vi "Analyze Fell Rocks.vi"(0 "Rock Position in Chamber in":i32=3, 1 "Push List":cluster{u8, i32}[](array[cluster]), 2 "Chamber":u32[][](array[colorbox]), 3 "Rock Settled ?":bool, 4 "Initialize ? (F)":bool) -> (5 "#Rocks Settled":i32, 6 "Tower Height":u64, 7 "Sequence Analysis":T1, 9 "Tower Heights":map{i32, u64}(c390))   [LabVIEW 2020, in "AoC 2022.lvlib"]
uses:
  AoC 2022.lvlib
  Sequence Analysis.ctl
  <vilib>/Utility/miscctls.llb/LVMapReplaceAction.ctl
panel:
  out "Sequence Found ? out":bool
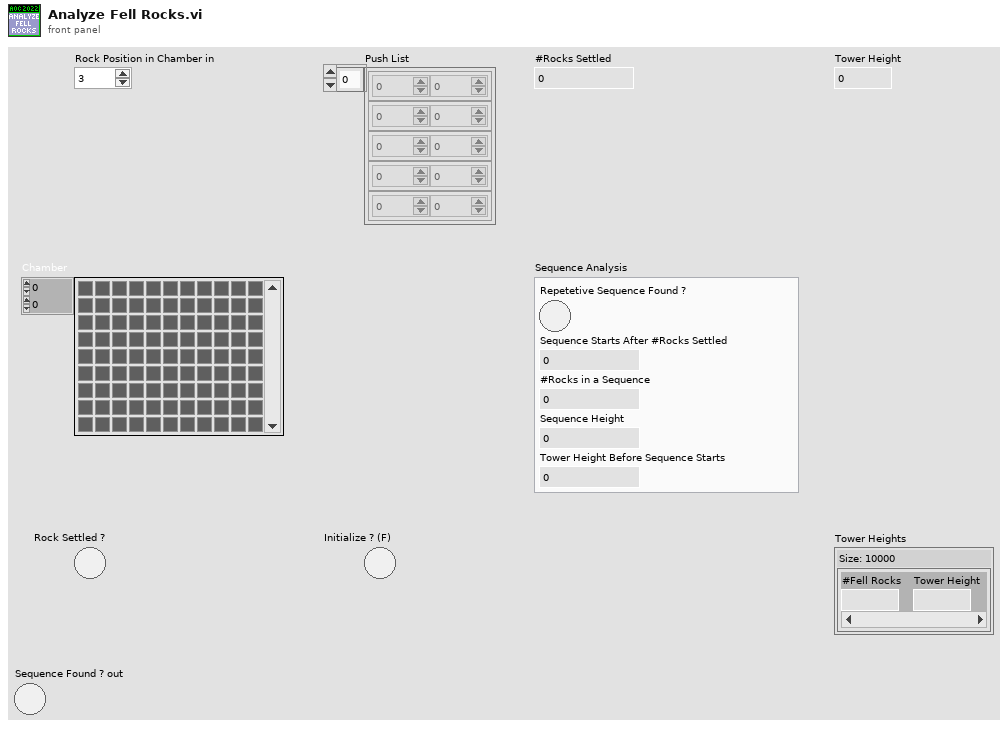
[diagram p1: front panel]
types:
  T1 = typedef "AoC 2022.lvlib/Sequence Analysis.ctl" = cluster{"Repetetive Sequence Found ?":bool, "Sequence Starts After #Rocks Settled":i32, "#Rocks in a Sequence":i32, "Sequence Height":u64, "Tower Height Before Sequence Starts":u64}
  T2 = map{cluster{"Chamber":u32[][], "Push Action":string}, i32[]}
  T3 = typedef "LVMapReplaceAction.ctl" = enum32{"Modify Entry only if found", "Add or Modify Entry", "Delete Entry"}
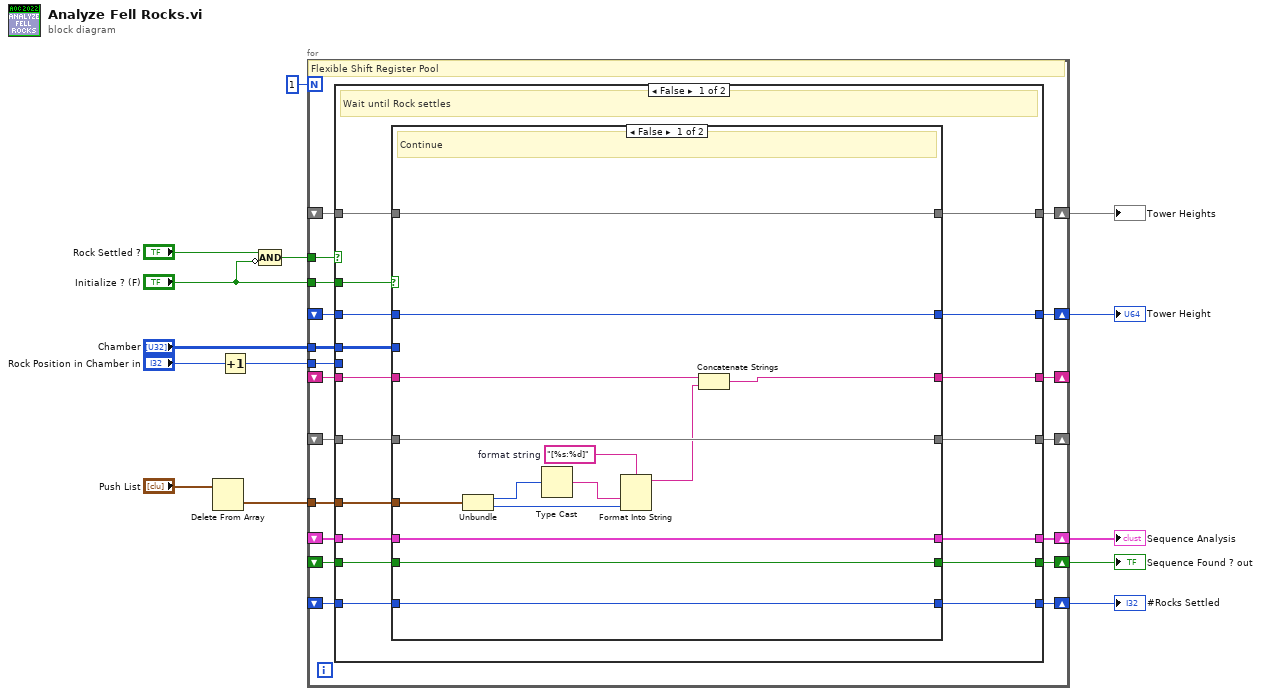
[diagram p0: block diagram]
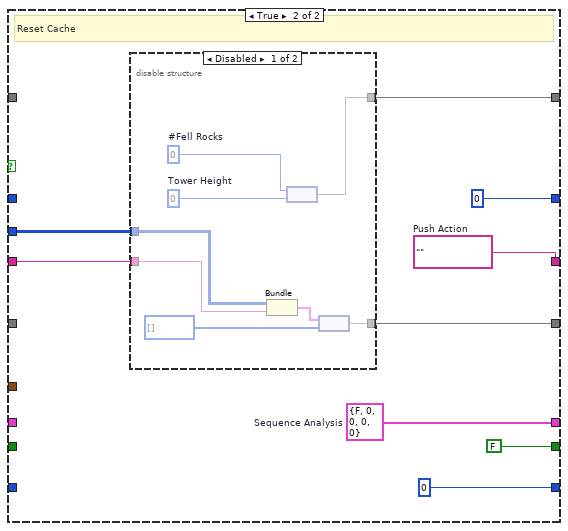
[diagram p2: hidden frame]
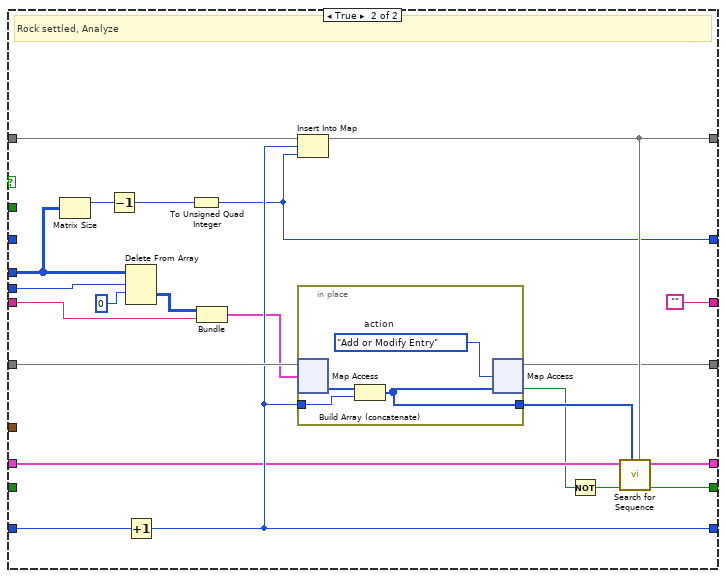
[diagram p4: hidden frame]
diagram:
  n1 = Delete From Array(array="Push List") -> (deleted portion=w6:cluster{u8, i32})  [unwired: 2 in, 1 out]
  n2 = Increment(x="Rock Position in Chamber in") -> (x+1=w4:i32)
  n3 = Compound Arithmetic op=AND("Rock Settled ?", invert "Initialize ? (F)") -> (w10:bool)
  n4 = for {
    N: 1 -> [_]
    tunnel: "Chamber" -> [w28]
    shift-right: [w29] -> _
    shift-left: _ -> [w33]
    tunnel: w10 -> [w32]
    shift-right: [w30] -> w11
    shift-left: _ -> [w31]
    tunnel: "Initialize ? (F)" -> [w27]
    shift-right: [w26] -> w3
    shift-left: _ -> [w25]
    shift-right: [w24] -> w2
    shift-left: _ -> [w23]
    shift-right: [w22] -> w9
    shift-left: _ -> [w21]
    tunnel: w6 -> [w20]
    shift-right: [w19] -> _
    shift-left: _ -> [w18]
    tunnel: w4 -> [w17]
    shift-right: [w16] -> w1
    shift-left: _ -> [w15]
    # "Flexible Shift Register Pool"
    n5 = case shown="False" w32 {
      tunnel: w33 -> [w46 w99]
      tunnel: w31 -> [w48 _]
      tunnel: [w49 w83] -> w30
      tunnel: [w47 w82] -> w29
      tunnel: w28 -> [w36 w98]
      tunnel: w27 -> [w50 _]
      tunnel: [w44 w103] -> w26
      tunnel: w25 -> [w45 w89]
      tunnel: [w42 w91] -> w24
      tunnel: w23 -> [w43 _]
      tunnel: [w41 w93] -> w22
      tunnel: w21 -> [w40 w100]
      tunnel: w20 -> [w39 _]
      tunnel: [w38 ""] -> w19
      tunnel: w18 -> [w37 w101]
      tunnel: w17 -> [_ w95]
      tunnel: [w35 w88] -> w16
      tunnel: w15 -> [w34 w94]
      frame False {
        # "Wait until Rock settles"
        n6 = case shown="False" w50 {
          tunnel: [w64 u64 0] -> w49
          tunnel: w48 -> [w64 _]
          tunnel: [w63 w65] -> w47
          tunnel: w46 -> [w63 _]
          tunnel: w45 -> [w62 _]
          tunnel: [w62 w66] -> w44
          tunnel: w43 -> [w61 _]
          tunnel: [w61 FALSE] -> w42
          tunnel: [w60 0] -> w41
          tunnel: w40 -> [w60 _]
          tunnel: w39 -> [w56 _]
          tunnel: [w59 w69] -> w38
          tunnel: w37 -> [w58 w71]
          tunnel: w36 -> [_ w68]
          tunnel: [w57 w67] -> w35
          tunnel: w34 -> [w57 _]
          frame False {
            w54 = "[%s:%d]"  # format string
            # "Continue"
            n7 = Unbundle(w56) -> (w55:u8, w52:i32)
            n8 = Type Cast(x=w55) -> (*(type *) &x=w53:string)  [unwired: 1 in]
            n9 = Format Into String(format string=w54, w53, w52) -> (resulting string=w51:string)  [unwired: 2 in, 1 out]
            n10 = Concatenate Strings(w58, w51) -> (w59:string)
          }
          frame True {
            w66 = T1 {"Repetetive Sequence Found ?"=FALSE, "Sequence Starts After #Rocks Settled"=0, "#Rocks in a Sequence"=0, "Sequence Height"=0, "Tower Height Before Sequence Starts"=0}  # Sequence Analysis
            w69 = ""  # Push Action
            # "Reset Cache"
            n11 = disable-structure shown="Disabled" {
              disable-tunnel: w71 -> [w80 _]
              disable-tunnel: [w79 _] -> w65
              disable-tunnel: w68 -> [w77 _]
              disable-tunnel: [w76 _] -> w67
              frame Disabled {
                w74 = u64 0  # Tower Height
                w75 = 0  # #Fell Rocks
                n12 = Bundle("Chamber"=w77, "Push Action"=w80) -> (w81:cluster{"Chamber":u32[][], "Push Action":string})  [unwired: 1 in]
                n13 = node(w75, w74) -> (w76:map{i32, u64})
                n14 = node(w81, i32[] [] ("Settled Rocks")) -> (w79:T2)
              }
              frame Enabled {
              }
            }
          }
        }
      }
      frame True {
        # "Rock settled, Analyze"
        n15 = Matrix Size(0:w98) -> (1:w102:i32)  [unwired: 1 out]
        n16 = Decrement(x=w102) -> (x-1=w92:i32)
        n17 = Delete From Array(array=w98, length=w95, index (row)=0) -> (deleted portion=w87:u32[][])  [unwired: 1 in, 1 out]
        n18 = Increment(x=w100) -> (x+1=w93:i32)
        n19 = To Unsigned Quad Integer(1:w92) -> (0:w83:u64)
        n20 = Bundle("Chamber"=w87, "Push Action"=w101) -> (w86:cluster{"Chamber":u32[][], "Push Action":string})  [unwired: 1 in]
        n21 = Insert Into Map(map in=w94, key=w93, value=w83) -> (map out=w88:map{i32, u64})  [unwired: 2 out]
        n22 = in-place {
          in-place-border: w93 -> [w106]
          in-place-border: [w104] -> w90
          w105 = LVMapReplaceAction."Add or Modify Entry"  # action
          n23 = in-place-map #1(w99, w86) -> (w107:i32[])  [unwired: 1 in, 1 out]
          n24 = Build Array (concatenate)(w107, w106) -> (w104:i32[])
          n25 = in-place-map #1(w104, w105) -> (w82:T2, w85:bool)  [unwired: 1 out]
        }
        n26 = Not(x=w85) -> (.not. x?=w84:bool)
        n27 = call "Search for Sequence.vi"("Tower Heights"=w88, "Settled Rocks"=w90, "Sequence Found ? in"=w84, "Sequence Analysis in"=w89) -> ("Sequence Found ? out"=w91:bool, "Sequence Analysis out"=w103:T1)  [unwired: 4 in]
      }
    }
  }
  "Tower Height" <- w11
  "#Rocks Settled" <- w9
  "Sequence Analysis" <- w3
  "Sequence Found ? out" <- w2
  "Tower Heights" <- w1
